vi "StartStop_nano.vi"(10 "STOP":bool, 11 "START":bool) -> ()   [LabVIEW 2019]
uses:
  Program Files/National Instruments/LabVIEW 2019/user.lib/HapticSTM/HapticSTM.lvlib
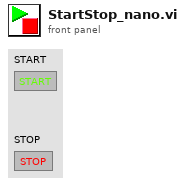
[diagram p1: front panel]
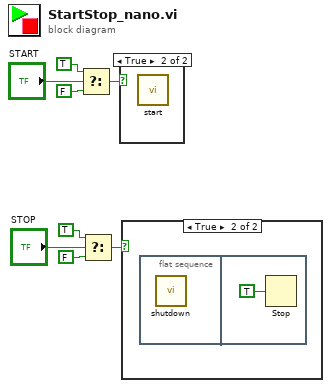
[diagram p0: block diagram]
diagram:
  n1 = Select(t=TRUE, s="START", f=FALSE) -> (s? t:f=w1:bool)
  n2 = Select(t=TRUE, s="STOP", f=FALSE) -> (s? t:f=w5:bool)
  n3 = case shown="True" w1 {
    frame False {
    }
    frame True {
      n4 = call "start.vi"() -> ()  [unwired: 11 in, 1 out]
    }
  }
  n5 = case shown="True" w5 {
    frame False {
    }
    frame True {
      n6 = flat-sequence {
        frame #0 {
          n7 = call "shutdown.vi"() -> ()  [unwired: 12 in]
        }
        frame #1 {
          n8 = Stop(stop? (T)=TRUE) -> ()
        }
      }
    }
  }
